vi "Read Data as BGR8 Image.vi"(7 "Alpha Channel Value (Default: 0)":u8, 8 "error in (no error)":errorcluster, 11 "Buffer in":refnum<class "Buffer.lvclass">) -> (0 "error out":errorcluster, 2 "Image":u32[][](array[numeric]), 3 "Buffer":refnum<class "Buffer.lvclass">)   [LabVIEW 2020, in "Buffer.lvclass"]
uses:
  Buffer.lvclass
  Buffer.lvclass/Buffer.ctl
  <vilib>/Utility/error.llb/Error Cluster From Error Code.vi
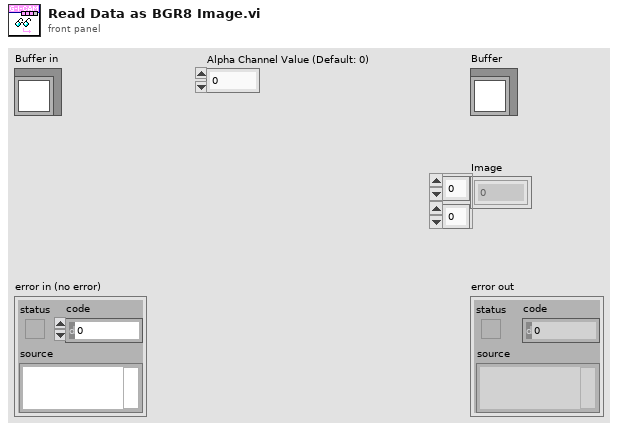
[diagram p1: front panel]
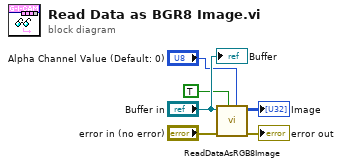
[diagram p0: block diagram]
diagram:
  n1 = call "ReadDataAsRGB8Image.vi"("alpha_channel_value"="Alpha Channel Value (Default: 0)", "Flip RB Channel Order"=TRUE, "error in (no error)"="error in (no error)", "Buffer in"="Buffer in") -> ("error out"=→"error out":errorcluster, "image"=→"Image":u32[][])  [unwired: 6 in]
  "Buffer" <- "Buffer in"
